vi "Stage State Machine.vi"(0 "Stage Button":bool, 1 "Stage Sensor":bool, 2 "Intake Sensor":bool) -> (3 "Stage Motor":T1, 4 "Intake Motor":T1, 5 "Flipper":enum16{"Closed", "Open"}(ring), 6 "Stage_Active":bool)   [LabVIEW 2015]
uses:
  Motor_Dir_Type_Def.ctl
  Stage_Type_Def.ctl
panel:
  in  "DB_Count":dbl
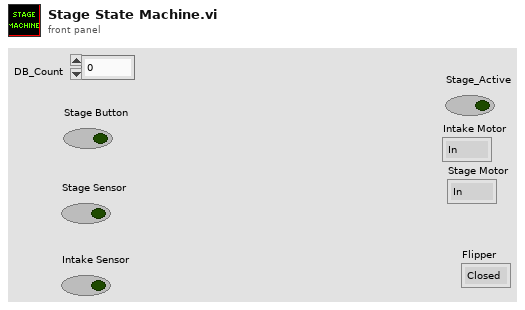
[diagram p1: front panel]
types:
  T1 = typedef "Motor_Dir_Type_Def.ctl" = enum16{"In", "Out", "Off"}
  T2 = typedef "Stage_Type_Def.ctl" = enum16{"Off", "Stage Intake", "Ball Stage", "Ball_Not_Found"}
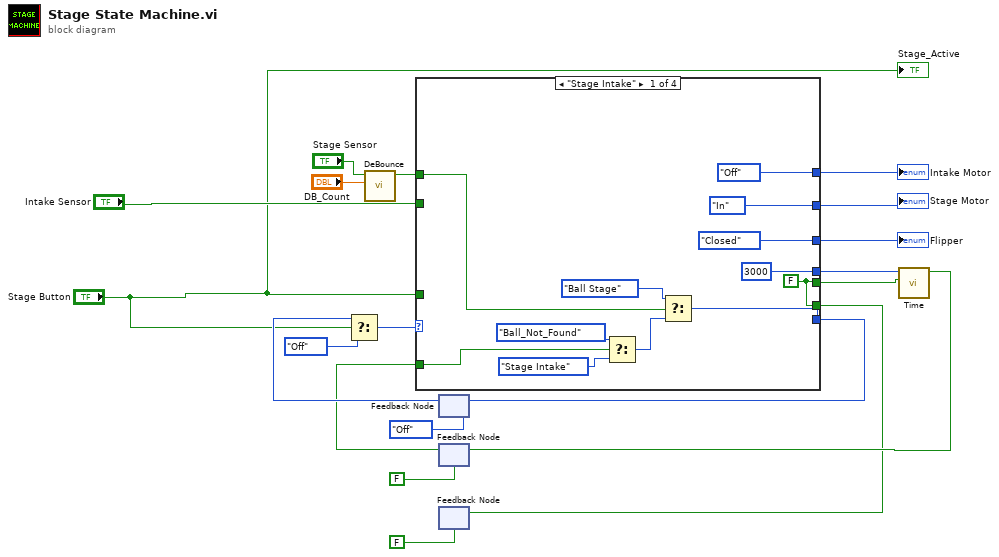
[diagram p0: block diagram]
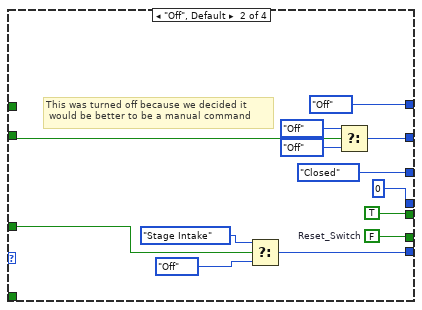
[diagram p2: hidden frame]
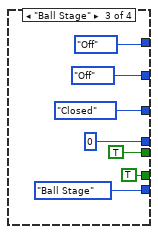
[diagram p3: hidden frame]
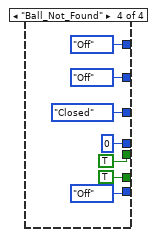
[diagram p4: hidden frame]
diagram:
  n1 = call "DeBounce.vi"("DB_Count"="DB_Count", "Value"="Stage Sensor") -> ("BD_Value"=w10:bool)  [unwired: 9 in]
  n2 = feedback #1(Stage_Type_Def."Off" ("Enum")) -> (w20:T2)
  n3 = Select(t=w20, s="Stage Button", f=Stage_Type_Def."Off" ("Enum")) -> (s? t:f=w19:T2)
  n4 = feedback #2(FALSE) -> (w6:bool)
  n5 = case shown="\"Stage Intake\"" w19 {
    tunnel: [w22 w45 Stage_Type_Def."Ball Stage" ("Enum") Stage_Type_Def."Off" ("Enum")] -> w18
    tunnel: "Stage Button" -> [_ w33 _ _]
    tunnel: [Motor_Dir_Type_Def."Off" ("Motor") Motor_Dir_Type_Def."Off" ("Motor") Motor_Dir_Type_Def."Off" ("Motor") Motor_Dir_Type_Def."Off" ("Motor")] -> w14
    tunnel: [Motor_Dir_Type_Def."In" ("Motor") w43 Motor_Dir_Type_Def."Off" ("Motor") Motor_Dir_Type_Def."Off" ("Motor")] -> w13
    tunnel: "Intake Sensor" -> [_ w44 _ _]
    tunnel: [enum16{"Closed", "Open"}."Closed" ("Enum") enum16{"Closed", "Open"}."Closed" ("Enum") enum16{"Closed", "Open"}."Closed" ("Enum") enum16{"Closed", "Open"}."Closed" ("Enum")] -> w15
    tunnel: w10 -> [w24 _ _ _]
    tunnel: [w27 TRUE TRUE TRUE] -> w7
    tunnel: [3000 0 0 0] -> w9
    tunnel: [w27 w34 TRUE TRUE ("Reset_Switch")] -> w2
    tunnel: w6 -> [w23 _ _ _]
    frame "Stage Intake" {
      w27 = FALSE
      n6 = Select(t=Stage_Type_Def."Ball_Not_Found" ("Enum"), s=w23, f=Stage_Type_Def."Stage Intake" ("Enum")) -> (s? t:f=w26:T2)
      n7 = Select(t=Stage_Type_Def."Ball Stage" ("Enum"), s=w24, f=w26) -> (s? t:f=w22:T2)
    }
    frame "Off", Default {
      w34 = FALSE  # Reset_Switch
      # "This was turned off because we decided it\n would be better to be a manual command"
      n8 = Select(t=Stage_Type_Def."Stage Intake" ("Enum"), s=w33, f=Stage_Type_Def."Off" ("Enum")) -> (s? t:f=w45:T2)
      n9 = Select(t=Motor_Dir_Type_Def."Off" ("Motor"), s=w44, f=Motor_Dir_Type_Def."Off" ("Motor")) -> (s? t:f=w43:T1)
    }
    frame "Ball Stage" {
    }
    frame "Ball_Not_Found" {
    }
  }
  "Flipper" <- w15
  "Intake Motor" <- w14
  "Stage Motor" <- w13
  n10 = feedback-in #1(w18) -> ()
  n11 = feedback #3(FALSE) -> ()  [unwired: 1 in]
  n12 = feedback-in #3(w2) -> ()
  n13 = call "Time.vi"("Reset"=w7, "Time_Limit  (ms)"=w9) -> ("Time_Met"=w4:bool)  [unwired: 9 in]
  n14 = feedback-in #2(w4) -> ()
  "Stage_Active" <- "Stage Button"
